vi "HB_ThreadPool.MainEventListenerTask.vi"() -> ()   [LabVIEW 2009, in "HB_BaseClass_Examples.lvlib"]
doc: "Simple application to test the HGF_ThreadPool with a simple class."
uses:
  HB_BaseClass_Examples.lvlib
  HB_Factory/HB_Factory.lvclass
  lib.lib/HGF_LVC/HGF_BaseClasses/HGF_Factory/HGF_Factory.lvclass
  lib.lib/HGF_LVC/HGF_BaseClasses/HGF_Event/HGF_Event.lvclass
  lib.lib/HGF_LVC/HGF_BaseClasses/HGF_ThreadTask/HGF_ThreadTask.lvclass
  HB_Simple/HB_Simple.lvclass
  lib.lib/HGF_LVC/HGF_BaseClasses/HGF_Queue/HGF_Queue.lvclass
  lib.lib/HGF_LVC/HGF_ObjectManager/HGF_OMFactory/HGF_OMFactory.lvclass
  lib.lib/HGF_LVC/HGF_BaseClasses/HGF_Stop/HGF_Stop.lvclass
  lib.lib/HGF_LVC/HGF_BaseClasses/HGF_ThreadPool/HGF_ThreadPool.lvclass
  lib.lib/HGF_LVC/HGF_BaseClasses/HGF_Reference/HGF_Reference.lvclass
  lib.lib/HGF_LVC/HGF_Auxiliary/HGF_Auxiliary.lvlib
  lib.lib/HGF_LVC/HGF_ObjectManager/HGF_ObjectManager.lvlib
  lib.lib/HGF_LVC/HGF_BaseClasses/HGF_Visitor/HGF_Visitor.lvclass
panel:
  in  "Increment":bool
  out "objectName":string
  in  "nofObjects":i32=10
  out "Waveform Chart":dbl(graph)
  in  "timeout in ms (-1)":i32=3000
  out "nofTasksInQueueOut":i32
  out "nofTasksWaiting":i32
  out "autoIncrementLimit":i32=-1
  out "nofThreads":i32
  out "Default Destination timed out?":bool
  out "got object?":bool
  out "error":errorcluster
  in  "stop":bool
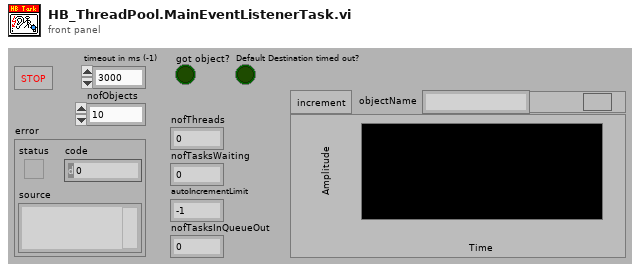
[diagram p1: front panel]
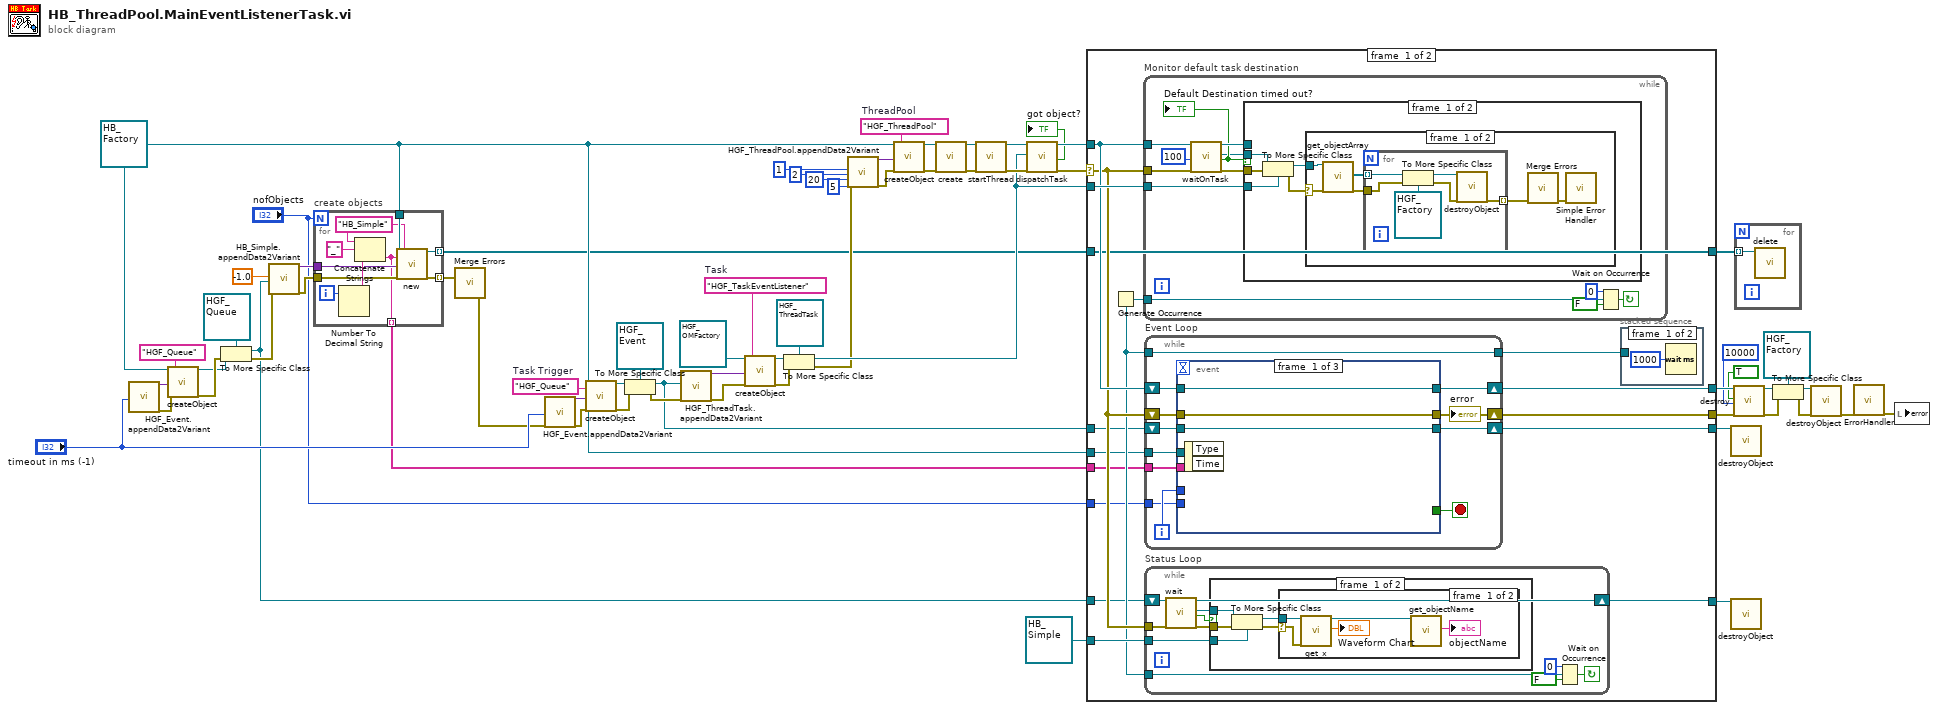
[diagram p0: block diagram]
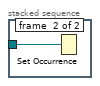
[diagram p2: hidden frame]
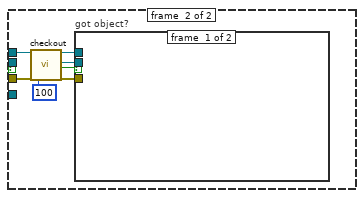
[diagram p6: hidden frame]
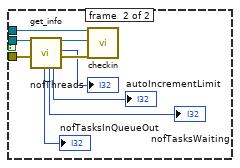
[diagram p7: hidden frame]
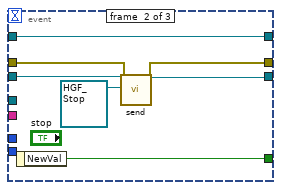
[diagram p8: hidden frame]
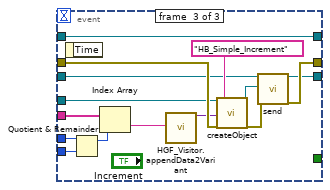
[diagram p9: hidden frame]
diagram:
  w48 = "HGF_Queue"  # Task Trigger
  w47 = "HGF_TaskEventListener"  # Task
  w40 = "HGF_ThreadPool"  # ThreadPool
  w21 = refnum<class "HB_Factory.lvclass"> refnum ("HB_Factory.lvclass")
  n1 = call "HGF_Event.appendData2Variant.vi"("timeout in ms (-1)"="timeout in ms (-1)") -> ("dup initData"=w25:variant, "error out"=w26:errorcluster)  [unwired: 2 in, 15 out]
  n2 = call "createObject.vi"("HGF_Factory"=w21, "initializationData"=w25, "error in (no error)"=w26, "className"="HGF_Queue") -> ("HGF_Object"=w22:refnum<class "HGF_Factory.lvclass">, "error out"=w23:errorcluster)  [unwired: 2 in, 12 out]
  n3 = To More Specific Class(target class=refnum<class "HGF_Queue.lvclass"> refnum ("HGF_BaseClasses.lvlib:HGF_Queue.lvclass"), reference=w22, error in=w23) -> (specific class reference=w14:refnum<class "HGF_Queue.lvclass">, error out=w15:errorcluster)
  n4 = call "HB_Simple.appendData2Variant.vi"("x"=-1.0, "statusEvent"=w14, "error in (no error)"=w15) -> ("dup initData"=w17:variant, "error out"=w16:errorcluster)  [unwired: 15 in]
  n5 = for "create objects" {
    N: "nofObjects" -> [_]
    tunnel: [w69] -> w7 mode=indexing
    tunnel: w21 -> [w71]
    tunnel: [w68] -> w12 mode=indexing
    tunnel: w17 -> [w73]
    tunnel: w16 -> [w72]
    tunnel: [w67] -> w3 mode=indexing
    i -> [w75]
    w70 = "HB_Simple" ("className")
    n6 = Number To Decimal String(number=w75) -> (decimal integer string=w74:string)  [unwired: 1 out]
    n7 = Concatenate Strings(w70, "_" ("string"), w74) -> (w67:string)
    n8 = call "new.vi"("HGF_Factory"=w71, "objectName"=w67, "initializationData"=w73, "error in (no error)"=w72, "className"=w70) -> ("objectRef"=w69:refnum<class "HGF_Reference.lvclass">, "error out"=w68:errorcluster)  [unwired: 4 in, 9 out]
  }
  n9 = call <vilib>:"Merge Errors.vi"("error array in"=w12) -> ("error out"=w6:errorcluster)  [unwired: 3 in, 3 out]
  n10 = call "HGF_Event.appendData2Variant.vi"("timeout in ms (-1)"="timeout in ms (-1)", "error in (no error)"=w6) -> ("dup initData"=w53:variant, "error out"=w52:errorcluster)  [unwired: 2 in, 14 out]
  n11 = call "createObject.vi"("HGF_Factory"=w21, "initializationData"=w53, "error in (no error)"=w52, "className"=w48) -> ("HGF_Object"=w45:refnum<class "HGF_Factory.lvclass">, "error out"=w54:errorcluster)  [unwired: 2 in, 12 out]
  n12 = To More Specific Class(target class=refnum<class "HGF_Event.lvclass"> refnum ("HGF_BaseClasses.lvlib:HGF_Event.lvclass"), reference=w45, error in=w54) -> (specific class reference=w28:refnum<class "HGF_Event.lvclass">, error out=w39:errorcluster)
  n13 = call "HGF_ThreadTask.appendData2Variant.vi"("taskTrigger"=w28, "error in (no error)"=w39) -> ("dup initData"=w37:variant, "error out"=w36:errorcluster)  [unwired: 4 in, 12 out]
  n14 = call "createObject.vi"("HGF_Factory"=refnum<class "HGF_OMFactory.lvclass"> refnum ("HGF_ObjectManager.lvlib:HGF_OMFactory.lvclass"), "initializationData"=w37, "error in (no error)"=w36, "className"=w47) -> ("HGF_Object"=w44:refnum<class "HGF_Factory.lvclass">, "error out"=w51:errorcluster)  [unwired: 2 in, 12 out]
  n15 = To More Specific Class(target class=refnum<class "HGF_ThreadTask.lvclass"> refnum ("HGF_BaseClasses.lvlib:HGF_ThreadTask.lvclass"), reference=w44, error in=w51) -> (specific class reference=w29:refnum<class "HGF_ThreadTask.lvclass">, error out=w18:errorcluster)
  n16 = call "HGF_ThreadPool.appendData2Variant.vi"("initialNofThreads (0)"=1 ("initialNofThreads"), "incThreads(1)"=2 ("incThreads"), "maxNofThreads (-1:unlimited)"=20 ("maxNofThreads"), "error in (no error)"=w18, "autoIncrementLimit (-1)"=5) -> ("dup initData"=w65:variant, "error out"=w19:errorcluster)  [unwired: 2 in, 11 out]
  n17 = call "createObject.vi"("HGF_Factory"=w21, "initializationData"=w65, "error in (no error)"=w19, "className"=w40) -> ("HGF_Object"=w46:refnum<class "HGF_Factory.lvclass">, "error out"=w64:errorcluster)  [unwired: 2 in, 12 out]
  n18 = call "create.vi"("Object"=w46, "error in (no error)"=w64) -> ("HGF_Reference"=w66:refnum<class "HGF_Reference.lvclass">, "error out"=w60:errorcluster)  [unwired: 1 in, 15 out]
  n19 = call "startThread.vi"("HGF_ThreadPool_Reference"=w66, "error in (no error)"=w60) -> ("dup HGF_ThreadPool_Reference"=w34:refnum<class "HGF_Reference.lvclass">, "error out"=w32:errorcluster)  [unwired: 1 in, 15 out]
  n20 = call "dispatchTask.vi"("HGF_ThreadPool_Reference"=w34, "HGF_ThreadTask"=w29, "error in (no error)"=w32) -> ("dup HGF_ThreadPool_Reference"=w33:refnum<class "HGF_Reference.lvclass">, "got object?"=→"got object?":bool, "error out"=w31:errorcluster)  [unwired: 1 in, 13 out]
  n21 = case shown="No Error" w31 {
    selector: w31 -> [w87 w201]
    tunnel: w33 -> [w89 w202]
    tunnel: [w92 w202] -> w50
    tunnel: w29 -> [w90 _]
    tunnel: [w91 w201] -> w49
    tunnel: w28 -> [w82 w199]
    tunnel: w14 -> [w83 w200]
    tunnel: refnum<class "HB_Simple.lvclass"> refnum ("HGF_BaseClass_Examples.lvlib:HB_Simple.lvclass") -> [w86 _]
    tunnel: w21 -> [w84 _]
    tunnel: [w81 w200] -> w9
    tunnel: [w80 w199] -> w8
    tunnel: w7 -> [w79 w198]
    tunnel: [w79 w198] -> w5
    tunnel: "nofObjects" -> [w78 _]
    tunnel: w3 -> [w77 _]
    frame #0 {
      n22 = Generate Occurrence() -> (w85:refnum<k4>)
      n23 = while "Monitor default task destination" {
        tunnel: w90 -> [w123]
        tunnel: w89 -> [w122]
        tunnel: w87 -> [w121]
        tunnel: w85 -> [w116]
        stop <- w117 continue-if-true
        n24 = call "waitOnTask.vi"("HGF_ThreadPool_Reference"=w122, "timeout in ms (-1)"=100, "error in (no error)"=w121) -> ("dup HGF_ThreadPool_Reference"=w127:refnum<class "HGF_Reference.lvclass">, "HGF_Task"=w125:refnum<class "HGF_ThreadTask.lvclass">, "timed out?"=w126:bool, "error out"=w120:errorcluster)  [unwired: 13 out]
        "Default Destination timed out?" <- w126
        n25 = case "timed out?" shown="True" w126 {
          tunnel: w125 -> [w132 _]
          tunnel: w120 -> [w131 w145]
          tunnel: w127 -> [_ w146]
          tunnel: w123 -> [w128 _]
          frame #0 {
            n26 = To More Specific Class(target class=w128, reference=w132, error in=w131) -> (specific class reference=w130:refnum<class "HGF_ThreadTask.lvclass">, error out=w129:errorcluster)
            n27 = case shown="No Error" w129 {
              selector: w129 -> [w137 _]
              tunnel: w130 -> [w138 _]
              frame #0 {
                n28 = call "get_objectArray.vi"("HGF_ThreadTask"=w138, "error in (no error)"=w137) -> ("objectArray"=w133:refnum<class>[], "error out"=w135:errorcluster)  [unwired: 16 out]
                n29 = for {
                  tunnel: w135 -> [w140]
                  tunnel: [w144] -> w136 mode=indexing
                  tunnel: w133 -> [w143] mode=indexing
                  n30 = To More Specific Class(target class=refnum<class "HGF_Factory.lvclass"> refnum ("HGF_BaseClasses.lvlib:HGF_Factory.lvclass"), reference=w143, error in=w140) -> (specific class reference=w142:refnum<class "HGF_Factory.lvclass">, error out=w141:errorcluster)
                  n31 = call "destroyObject.vi"("HGF_Factory"=w142, "error in (no error)"=w141) -> ("error out"=w144:errorcluster)  [unwired: 17 out]
                }
                n32 = call <vilib>:"Merge Errors.vi"("error array in"=w136) -> ("error out"=w134:errorcluster)  [unwired: 3 in, 3 out]
                n33 = call <vilib>:"Simple Error Handler.vi"("error in (no error)"=w134) -> ()  [unwired: 1 in, 8 out]
              }
              frame #1 {
              }
            }
          }
          frame #1 {
            n34 = call "checkout.vi"("HGF_ThreadPool_Reference"=w146, "timeout in ms (-1)"=100, "error in (no error)"=w145) -> ("dup HGF_ThreadPool_Reference"=w147:refnum<class "HGF_Reference.lvclass">, "HGF_ThreadPool"=w148:refnum<class "HGF_ThreadPool.lvclass">, "got object?"=w151:bool, "error out"=w149:errorcluster)  [unwired: 13 out]
            n35 = case "got object?" shown="True" w151 {
              tunnel: w147 -> [_ w160]
              tunnel: w148 -> [_ w159]
              tunnel: w149 -> [_ w158]
              frame #0 {
              }
              frame #1 {
                n36 = call "get_info.vi"("HGF_ThreadPool"=w159, "error in (no error)"=w158) -> ("nofTasksInQueueOut"=→"nofTasksInQueueOut":i32, "nofTasksWaiting"=→"nofTasksWaiting":i32, "autoIncrementLimit"=→"autoIncrementLimit":i32, "dup HGF_ThreadPool"=w156:refnum<class "HGF_ThreadPool.lvclass">, "nofThreads"=→"nofThreads":i32, "error out"=w157:errorcluster)  [unwired: 12 out]
                n37 = call "checkin.vi"("HGF_Reference"=w160, "Object"=w156, "error in (no error)"=w157) -> ()  [unwired: 1 in, 16 out]
              }
            }
          }
        }
        n38 = Wait on Occurrence(1:FALSE ("ignore previous (T)"), 2:w116, 3:0 ("ms timeout (-1)")) -> (0:w117:bool)
      }
      n39 = while "Event Loop" {
        shift-right: [w171] -> w92
        shift-left: w89 -> [w170]
        shift-right: [w161] -> w91
        shift-left: w87 -> [w172]
        tunnel: w85 -> [w167]
        tunnel: [w167] -> w88
        tunnel: w84 -> [w168]
        shift-right: [w165] -> w80
        shift-left: w82 -> [w169]
        tunnel: w78 -> [w163]
        tunnel: w77 -> [w162]
        i -> [w164]
        stop <- w166 stop-if-true
        n40 = event shown="[2] \"Increment\": Value Change" {
          selector: _ -> [_ _ _]
          dyn-events: _ -> [_ _ _]
          timeout: _ -> [_ _ _]
          tunnel: [_ w182 _] -> w166
          tunnel: [w174 w177 w191] -> w161
          tunnel: w172 -> [w174 w178 w195]
          tunnel: [w175 w181 w197] -> w171
          tunnel: w170 -> [w175 w181 w197]
          tunnel: w169 -> [w173 w180 w194]
          tunnel: w168 -> [_ _ w190]
          tunnel: [w173 w176 w189] -> w165
          tunnel: w164 -> [_ _ w187]
          tunnel: w163 -> [_ _ w186]
          tunnel: w162 -> [_ _ w185]
          event #0 {
            n41 = event-data() -> ()  [unwired: 3 out]
          }
          event #1 {
            n42 = event-data() -> ("NewVal"=w182:bool)  [unwired: 1 out]
            n43 = call-dynamic "send.vi"("HGF_Event"=w180, "Object"=refnum<class "HGF_Stop.lvclass"> refnum ("HGF_BaseClasses.lvlib:HGF_Stop.lvclass"), "error in (no error)"=w178) -> ("dup HGF_Event"=w176:refnum<class "HGF_Event.lvclass">, "error out"=w177:errorcluster)  [unwired: 2 in, 13 out]
          }
          event #2 {
            n44 = event-data() -> ()  [unwired: 2 out]
            n45 = Quotient & Remainder(x=w187, y=w186) -> (x-y*floor(x/y)=w184:i32)  [unwired: 1 out]
            n46 = Index Array(array=w185, index=w184) -> (element=w183:string)
            n47 = call "HGF_Visitor.appendData2Variant.vi"("addressee"=w183) -> ("dup initData"=w188:variant)  [unwired: 3 in, 15 out]
            n48 = call "createObject.vi"("HGF_Factory"=w190, "initializationData"=w188, "error in (no error)"=w195, "className"="HB_Simple_Increment") -> ("HGF_Object"=w193:refnum<class "HGF_Factory.lvclass">, "error out"=w192:errorcluster)  [unwired: 2 in, 12 out]
            n49 = call-dynamic "send.vi"("HGF_Event"=w194, "Object"=w193, "error in (no error)"=w192) -> ("dup HGF_Event"=w189:refnum<class "HGF_Event.lvclass">, "error out"=w191:errorcluster)  [unwired: 2 in, 13 out]
          }
        }
        "error" <- w161
      }
      n50 = while "Status Loop" {
        tunnel: w87 -> [w104]
        tunnel: w86 -> [w101]
        tunnel: w85 -> [w96]
        shift-right: [w95] -> w81
        shift-left: w83 -> [w105]
        stop <- w97 continue-if-true
        n51 = call-dynamic "wait.vi"("HGF_Queue"=w105, "error in (no error)"=w104) -> ("dup HGF_Queue"=w95:refnum<class "HGF_Queue.lvclass">, "Object"=w102:refnum<class>, "timed out"=w100:bool, "error out"=w103:errorcluster)  [unwired: 2 in, 12 out]
        n52 = case shown="True" w100 {
          tunnel: w103 -> [w110 _]
          tunnel: w102 -> [w109 _]
          tunnel: w101 -> [w108 _]
          frame #0 {
            n53 = To More Specific Class(target class=w108, reference=w109, error in=w110) -> (specific class reference=w106:refnum<class "HB_Simple.lvclass">, error out=w107:errorcluster)
            n54 = case shown="No Error" w107 {
              selector: w107 -> [w114 _]
              tunnel: w106 -> [w115 _]
              frame #0 {
                n55 = call "get_x.vi"("HB_Simple"=w115, "error in (no error)"=w114) -> ("dup HB_Simple"=w112:refnum<class "HB_Simple.lvclass">, "x"=→"Waveform Chart":dbl)  [unwired: 16 out]
                n56 = call "get_objectName.vi"("HGF_Factory"=w112) -> ("objectName"=→"objectName":string)  [unwired: 1 in, 17 out]
              }
              frame #1 {
              }
            }
          }
          frame #1 {
          }
        }
        n57 = Wait on Occurrence(1:FALSE ("ignore previous (T)"), 2:w96, 3:0 ("ms timeout (-1)")) -> (0:w97:bool)
      }
      n58 = stacked-sequence {
        tunnel: w88 -> [_ w94]
        frame #0 {
          n59 = Wait (ms)(milliseconds to wait=u32 1000) -> ()  [unwired: 1 out]
        }
        frame #1 {
          n60 = Set Occurrence(w94) -> ()
        }
      }
    }
    frame #1 {
    }
  }
  n61 = call "destroyObject.vi"("HGF_Factory"=w8) -> ()  [unwired: 1 in, 18 out]
  n62 = call "destroyObject.vi"("HGF_Factory"=w9) -> ()  [unwired: 1 in, 18 out]
  n63 = call "destroy.vi"("HGF_Reference"=w50, "wait for activity? (F)"=TRUE, "timeout /ms (-1)"=10000, "error in (no error)"=w49) -> ("Object"=w59:refnum<class>, "error out"=w57:errorcluster)  [unwired: 14 out]
  n64 = for {
    tunnel: w5 -> [w203] mode=indexing
    n65 = call "delete.vi"("objectRef"=w203) -> ()  [unwired: 3 in, 4 out]
  }
  n66 = To More Specific Class(target class=refnum<class "HGF_Factory.lvclass"> refnum ("HGF_BaseClasses.lvlib:HGF_Factory.lvclass"), reference=w59, error in=w57) -> (specific class reference=w58:refnum<class "HGF_Factory.lvclass">, error out=w56:errorcluster)
  n67 = call "destroyObject.vi"("HGF_Factory"=w58, "error in (no error)"=w56) -> ("error out"=w38:errorcluster)  [unwired: 17 out]
  n68 = call "ErrorHandler.vi"("error in (no error)"=w38) -> ("error out"=w2:errorcluster)  [unwired: 6 in, 12 out]
  n69 = local write "error"(w2) -> ()
